vi "CS Control Single.vi"() -> ()   [LabVIEW 2019]
panel:
  in  "Quit":bool
  out "ID":string
  in  "URL":refnum<visa-resource-name>="tcp://localhost"
  in  "Quit 2":bool
  in  "Float":bool
  in  "Enable":bool
  in  "X":dbl[unit](slide)
  # "CS Control"
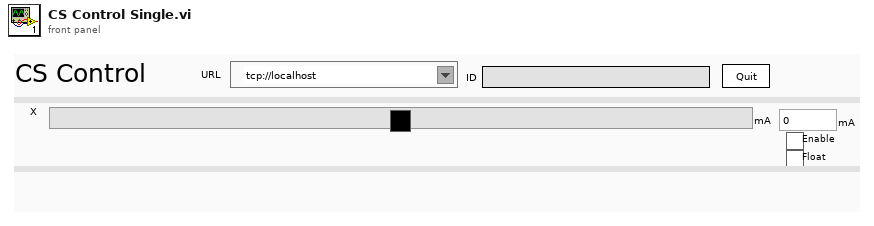
[diagram p1: front panel]
types:
  T1 = cluster{"TS Connection":cluster{"Type":enum16{"Serial", "TCP", "UDP", "mUDP"}, "URL":refnum<visa-resource-name>, "TO":u32, "Addr":u32, "Port":i32, "TCP":refnum<k5>, "UDP":refnum<k16>, "Route":string}, "REQ":refnum<queue>, "REP":refnum<queue>}
  T2 = cluster{"Awaiting REP":bool, "REQ ID":u32, "streams in":cluster{"id":u16, "timebase id":u16, "period":u32, "offset":u32, "sample number":u64, "total components":u16, "flags":u16, "components":cluster{"source id":u16, "flags":u16, "period":u32, "offset":u32}[]}[], "sources":cluster{"id":u16, "timebase_id":u16, "period":u32, "offset":u32, "fmt":i32, "flags":u16, "channels":u16, "type":u8, "name":string, "column names":string[], "title":string, "units":string}[], "timebases":cluster{"id":u16, "source":u8, "epoch":u8, "start time":u64, "period numerator (µs)":u32, "period denominator (µs)":u32, "flags":u32, "stability":sgl, "source id":string}[]}
  T3 = cluster{"TC Connection":cluster{"Type":enum16{"Serial", "TCP", "UDP", "mUDP"}, "URL":refnum<visa-resource-name>, "TO":u32, "Addr":u32, "Port":i32, "TCP":refnum<k5>, "UDP":refnum<k16>, "Route":string}, "REQ":refnum<queue>, "REP":refnum<queue>}
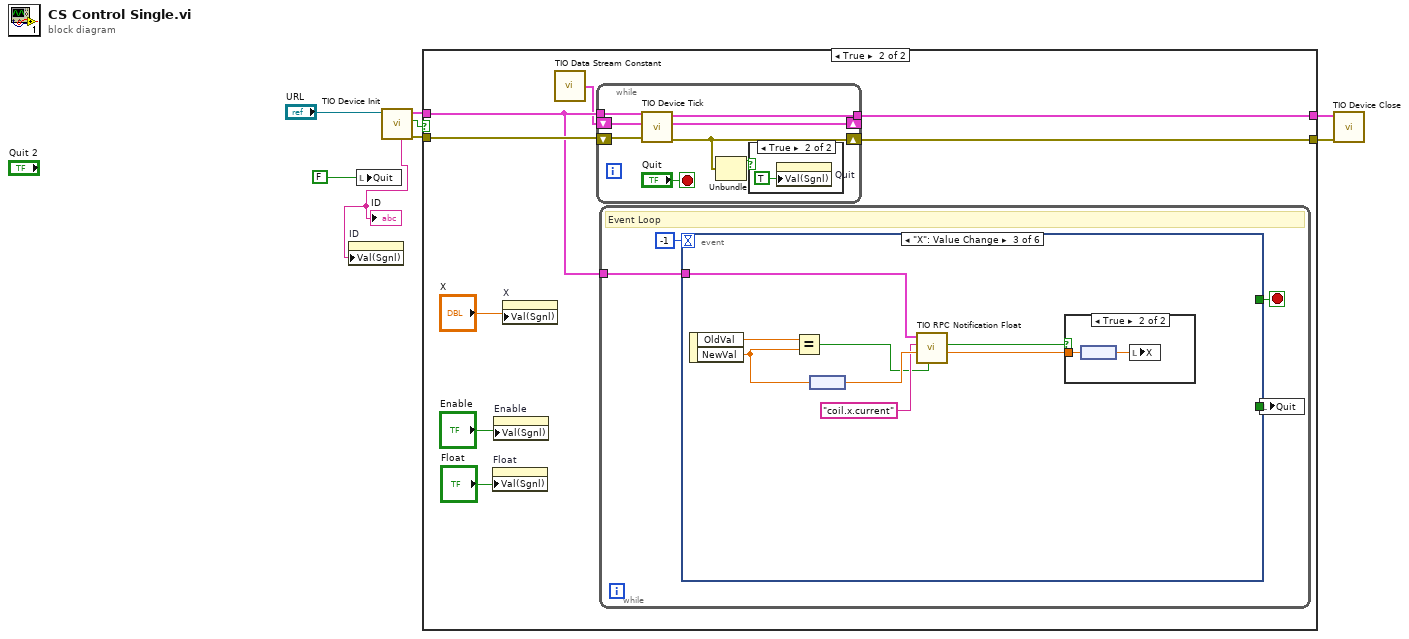
[diagram p0: block diagram]
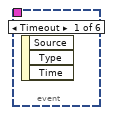
[diagram p4: hidden frame]
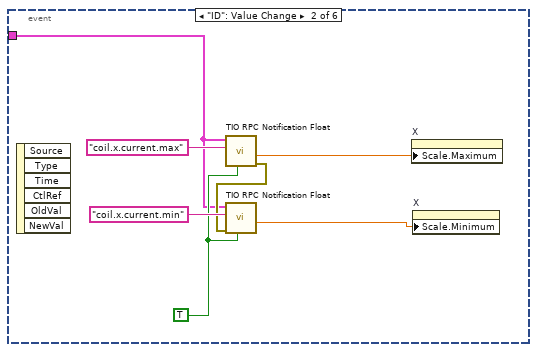
[diagram p5: hidden frame]
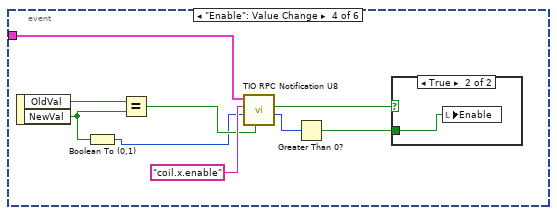
[diagram p7: hidden frame]
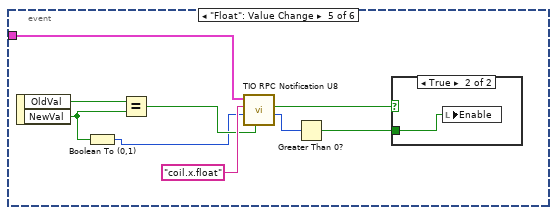
[diagram p9: hidden frame]
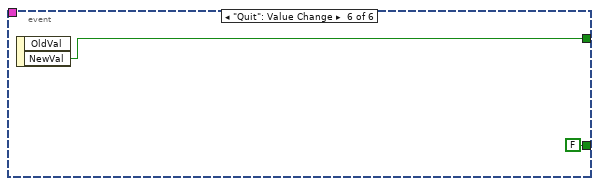
[diagram p11: hidden frame]
diagram:
  n1 = local write "Quit"(FALSE ("Quit")) -> ()
  n2 = call "TIO Device Init.vi"("URL"="URL") -> ("error out"=w5:errorcluster, 2:"ID Verified"=w6:bool, "TIO"=w7:T1, 4:"ID Verified"=w1:string)  [unwired: 6 in, 1 out]
  "ID" <- w1
  n3 = property on="ID" class="Str"("Val(Sgnl)"=w1) -> ()  [unwired: 2 in, 2 out]
  n4 = case shown="True" w6 {
    tunnel: w7 -> [w10 w16]
    tunnel: w5 -> [w9 w17]
    tunnel: [w9 w15] -> w3
    tunnel: [w10 w14] -> w2
    frame False {
    }
    frame True {
      n5 = property on="Float" class="Bool (strict)"("Val(Sgnl)"="Float") -> ()  [unwired: 2 in, 2 out]
      n6 = property on="Enable" class="Bool (strict)"("Val(Sgnl)"="Enable") -> ()  [unwired: 2 in, 2 out]
      n7 = property on="X" class="Slide (strict)"("Val(Sgnl)"="X") -> ()  [unwired: 2 in, 2 out]
      n8 = call "TIO Data Stream Constant.vi"() -> ("TIO State"=w13:T2)
      n9 = while {
        tunnel: w16 -> [w25]
        shift-right: [w23] -> _
        shift-left: w13 -> [w22]
        tunnel: [w21] -> w14
        shift-right: [w20] -> w15
        shift-left: w17 -> [w26]
        stop <- "Quit" stop-if-true
        n10 = call "TIO Device Tick.vi"("Error in"=w26, "TIO State"=w22, "TIO"=w25) -> ("Error out"=w20:errorcluster, "TIO State"=w23:T2, "TIO"=w21:T3)  [unwired: 5 in, 1 out]
        n11 = Unbundle(w20) -> ("status"=w19:bool)  [unwired: 2 out]
        n12 = case shown="True" w19 {
          frame False {
          }
          frame True {
            n13 = property on="Quit" class="Bool (strict)"("Val(Sgnl)"=TRUE ("Value (Signaling)")) -> ()  [unwired: 2 in, 2 out]
          }
        }
      }
      n14 = while {
        tunnel: w16 -> [w30]
        stop <- w29 stop-if-true
        # "Event Loop"
        n15 = event shown="[2] \"X\": Value Change" {
          selector: _ -> [_ _ _ _ _ _]
          dyn-events: _ -> [_ _ _ _ _ _]
          timeout: -1 -> [_ _ _ _ _ _]
          tunnel: w30 -> [_ w33 w41 w55 w65 _]
          tunnel: [_ _ _ _ _ w70] -> w29
          tunnel: [_ _ _ _ _ FALSE ("Quit")] -> w28
          event Timeout {
            n16 = event-data() -> ()  [unwired: 1 in, 3 out]
          }
          event "ID": Value Change {
            w34 = TRUE ("Read")
            n17 = event-data() -> ()  [unwired: 1 in, 6 out]
            n18 = call "TIO RPC Notification Float.vi"("Read"=w34, "Topic"="coil.x.current.max", "TIO"=w33) -> ("error out"=w35:errorcluster, "Get value (default if error)"=w36:sgl)  [unwired: 5 in, 1 out]
            n19 = call "TIO RPC Notification Float.vi"("Read"=w34, "error in (no error)"=w35, "Topic"="coil.x.current.min", "TIO"=w33) -> ("Get value (default if error)"=w32:sgl)  [unwired: 4 in, 2 out]
            n20 = property on="X" class="Slide (strict)"("Scale.Maximum"=w36) -> ()  [unwired: 2 in, 2 out]
            n21 = property on="X" class="Slide (strict)"("Scale.Minimum"=w32) -> ()  [unwired: 2 in, 2 out]
          }
          event "X": Value Change {
            n22 = event-data() -> ("OldVal"=w43:dbl[unit], "NewVal"=w42:dbl[unit])  [unwired: 1 in]
            n23 = Equal?(x=w43, y=w42) -> (x = y?=w39:bool)
            n24 = node(w42) -> (w46:dbl)
            n25 = call "TIO RPC Notification Float.vi"("Read"=w39, "Set value"=w46, "Topic"="coil.x.current", "TIO"=w41) -> ("Get value (default if error)"=w45:sgl, "Response"=w44:bool)  [unwired: 4 in, 1 out]
            n26 = case shown="True" w44 {
              tunnel: w45 -> [_ w48]
              frame False {
              }
              frame True {
                n27 = node(w48) -> (w47:sgl[unit])
                n28 = local write "X"(w47) -> ()
              }
            }
          }
          event "Enable": Value Change {
            n29 = event-data() -> ("OldVal"=w56:bool, "NewVal"=w52:bool)  [unwired: 1 in]
            n30 = Boolean To (0,1)(Boolean=w52) -> (0, 1=w51:i16)
            n31 = Equal?(x=w56, y=w52) -> (x = y?=w53:bool)
            n32 = call "TIO RPC Notification U8.vi"("Read"=w53, "U8"=w51, "Topic"="coil.x.enable", "TIO"=w55) -> ("U8"=w50:u8, "Response"=w57:bool)  [unwired: 4 in, 1 out]
            n33 = Greater Than 0?(x=w50) -> (x > 0?=w49:bool)
            n34 = case shown="True" w57 {
              tunnel: w49 -> [_ w58]
              frame False {
              }
              frame True {
                n35 = local write "Enable"(w58) -> ()
              }
            }
          }
          event "Float": Value Change {
            n36 = event-data() -> ("OldVal"=w66:bool, "NewVal"=w62:bool)  [unwired: 1 in]
            n37 = Boolean To (0,1)(Boolean=w62) -> (0, 1=w61:i16)
            n38 = Equal?(x=w66, y=w62) -> (x = y?=w63:bool)
            n39 = call "TIO RPC Notification U8.vi"("Read"=w63, "U8"=w61, "Topic"="coil.x.float", "TIO"=w65) -> ("U8"=w60:u8, "Response"=w67:bool)  [unwired: 4 in, 1 out]
            n40 = Greater Than 0?(x=w60) -> (x > 0?=w59:bool)
            n41 = case shown="True" w67 {
              tunnel: w59 -> [_ w68]
              frame False {
              }
              frame True {
                n42 = local write "Enable"(w68) -> ()
              }
            }
          }
          event "Quit": Value Change {
            n43 = event-data() -> ("NewVal"=w70:bool)  [unwired: 1 in, 1 out]
          }
        }
        n44 = local write "Quit"(w28) -> ()
      }
    }
  }
  n45 = call "TIO Device Close.vi"("Error in"=w3, "TIO"=w2) -> ()  [unwired: 10 in]
